vi "7. Producer Consumer Based Traffic Light Simulator.vi"() -> ()   [LabVIEW 2018]
uses:
  Typedefs/States for Producer Consumer Traffic Light.ctl
panel:
  in  "stop":bool
  out "Yellow":bool
  out "Green":bool
  out "Red":bool
  out "Traffic Lights Picture":picture
  # "Traffic Light Graphic Vector by Vecteezy\n(https://www.vecteezy.com/free-vector/graphic)"
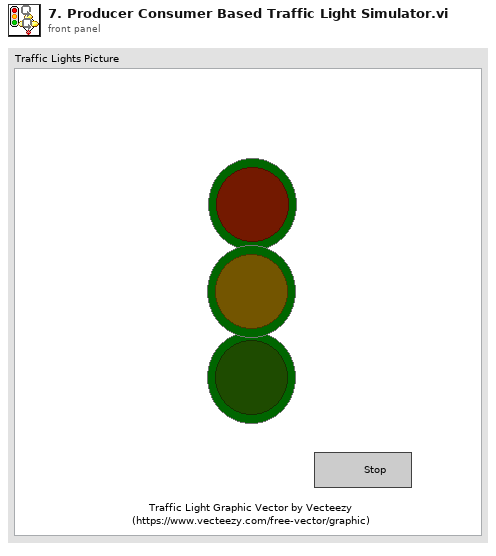
[diagram p1: front panel]
types:
  T1 = typedef "States for Producer Consumer Traffic Light.ctl" = enum16{"Red", "Yellow", "Green", "Stop"}
  T2 = cluster{"Wait Before Red":u32, "Wait Before Yellow":u32, "Wait Before Green":u32}
  T3 = cluster{"Wait Before Red":i32, "Wait Before Yellow":i32, "Wait Before Green":i32}
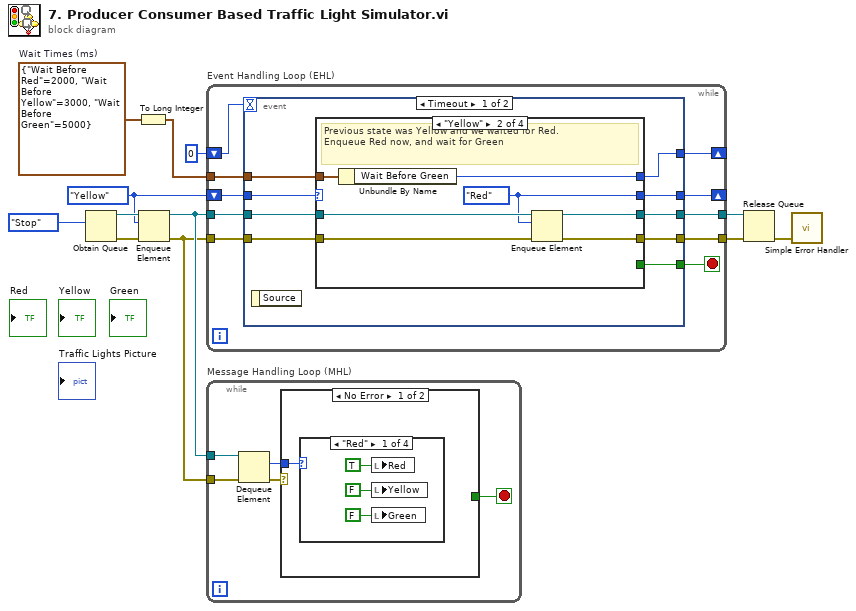
[diagram p0: block diagram]
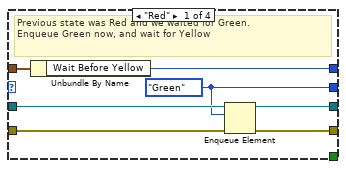
[diagram p2: hidden frame]
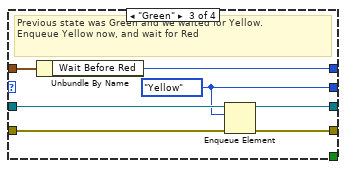
[diagram p3: hidden frame]
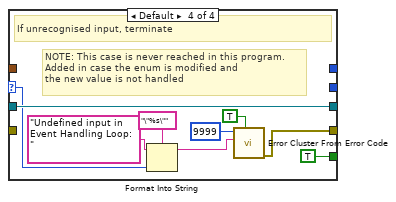
[diagram p4: hidden frame]
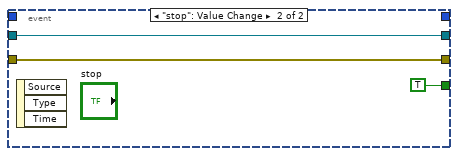
[diagram p5: hidden frame]
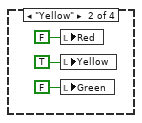
[diagram p6: hidden frame]
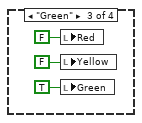
[diagram p7: hidden frame]
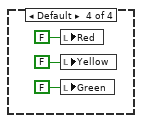
[diagram p8: hidden frame]
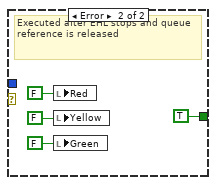
[diagram p9: hidden frame]
diagram:
  w2 = States_for_Producer_Consumer_Traffic_Light."Yellow" ("element")
  w11 = T2 {"Wait Before Red"=2000, "Wait Before Yellow"=3000, "Wait Before Green"=5000}  # Wait Times (ms)
  n1 = Obtain Queue(element data type=States_for_Producer_Consumer_Traffic_Light."Stop") -> (queue out=w12:refnum<queue>, error out=w7:errorcluster)  [unwired: 4 in, 1 out]
  n2 = To Long Integer(number=w11) -> (32bit integer=w9:T3)
  n3 = Enqueue Element(queue=w12, element=w2, error in (no error)=w7) -> (queue out=w8:refnum<queue>, error out=w6:errorcluster)  [unwired: 1 in, 1 out]
  n4 = while "Event Handling Loop (EHL)" {
    tunnel: w8 -> [w21]
    shift-right: [w16] -> _
    shift-left: w2 -> [w20]
    tunnel: w9 -> [w19]
    shift-right: [w15] -> _
    shift-left: 0 ("Wait Before Green") -> [w18]
    tunnel: [w17] -> w4
    tunnel: w6 -> [w14]
    tunnel: [w13] -> w5
    stop <- w22 stop-if-true
    n5 = event shown="[0] Timeout" {
      selector: _ -> [_ _]
      dyn-events: _ -> [_ _]
      timeout: w18 -> [_ _]
      tunnel: [w23 TRUE] -> w22
      tunnel: w21 -> [w31 w63]
      tunnel: w20 -> [w30 _]
      tunnel: w19 -> [w29 _]
      tunnel: [w28 _] -> w15
      tunnel: [w27 w63] -> w17
      tunnel: [w26 _] -> w16
      tunnel: w14 -> [w25 w62]
      tunnel: [w24 w62] -> w13
      event Timeout {
        n6 = event-data() -> ()  [unwired: 1 in, 1 out]
        n7 = case shown="\"Yellow\"" w30 {
          selector: w30 -> [_ _ _ w55]
          tunnel: w31 -> [w38 w45 w52 w61]
          tunnel: w29 -> [w37 w44 w51 _]
          tunnel: [w36 w43 w50 _] -> w28
          tunnel: [w35 w42 w49 w61] -> w27
          tunnel: [w34 w41 w48 _] -> w26
          tunnel: w25 -> [w33 w40 w47 _]
          tunnel: [w32 w39 w46 w59] -> w24
          tunnel: [_ _ _ TRUE] -> w23
          frame "Red" {
            w34 = States_for_Producer_Consumer_Traffic_Light."Green" ("element")
            # "Previous state was Red and we waited for Green.\nEnqueue Green now, and wait for Yellow"
            n8 = Unbundle By Name(w37) -> ("Wait Before Yellow"=w36:i32)
            n9 = Enqueue Element(queue=w38, element=w34, error in (no error)=w33) -> (queue out=w35:refnum<queue>, error out=w32:errorcluster)  [unwired: 1 in, 1 out]
          }
          frame "Yellow" {
            w41 = States_for_Producer_Consumer_Traffic_Light."Red" ("element")
            # "Previous state was Yellow and we waited for Red.\nEnqueue Red now, and wait for Green"
            n10 = Unbundle By Name(w44) -> ("Wait Before Green"=w43:i32)
            n11 = Enqueue Element(queue=w45, element=w41, error in (no error)=w40) -> (queue out=w42:refnum<queue>, error out=w39:errorcluster)  [unwired: 1 in, 1 out]
          }
          frame "Green" {
            w48 = States_for_Producer_Consumer_Traffic_Light."Yellow" ("element")
            # "Previous state was Green and we waited for Yellow.\nEnqueue Yellow now, and wait for Red"
            n12 = Unbundle By Name(w51) -> ("Wait Before Red"=w50:i32)
            n13 = Enqueue Element(queue=w52, element=w48, error in (no error)=w47) -> (queue out=w49:refnum<queue>, error out=w46:errorcluster)  [unwired: 1 in, 1 out]
          }
          frame Default {
            # "NOTE: This case is never reached in this program.\nAdded in case the enum is modified and\nthe new value is not handled"
            # "If unrecognised input, terminate"
            n14 = Format Into String(format string="\"%s\"", initial string="Undefined input in Event Handling Loop: " ("error message (\"\")"), w55) -> (resulting string=w54:string)  [unwired: 1 in, 1 out]
            n15 = call <vilib>:"Error Cluster From Error Code.vi"("show call chain? (False)"=TRUE, "error message (\"\")"=w54, "error code (0)"=9999) -> ("error out"=w59:errorcluster)  [unwired: 6 in]
          }
        }
      }
      event "stop": Value Change {
        n16 = event-data() -> ()  [unwired: 1 in, 3 out]
      }
    }
  }
  n17 = while "Message Handling Loop (MHL)" {
    tunnel: w8 -> [w68]
    tunnel: w6 -> [w66]
    stop <- w69 stop-if-true
    n18 = Dequeue Element(queue=w68, error in (no error)=w66) -> (element=w67:T1, error out=w65:errorcluster)  [unwired: 1 in, 2 out]
    n19 = case shown="No Error" w65 {
      tunnel: [_ TRUE] -> w69
      tunnel: w67 -> [w70 _]
      frame No Error {
        n20 = case shown="\"Red\"" w70 {
          frame "Red" {
            n21 = local write "Red"(TRUE ("Red")) -> ()
            n22 = local write "Yellow"(FALSE ("Red")) -> ()
            n23 = local write "Green"(FALSE ("Red")) -> ()
          }
          frame "Yellow" {
            n24 = local write "Red"(FALSE ("Red")) -> ()
            n25 = local write "Yellow"(TRUE ("Red")) -> ()
            n26 = local write "Green"(FALSE ("Red")) -> ()
          }
          frame "Green" {
            n27 = local write "Red"(FALSE ("Red")) -> ()
            n28 = local write "Yellow"(FALSE ("Red")) -> ()
            n29 = local write "Green"(TRUE ("Red")) -> ()
          }
          frame Default {
            n30 = local write "Red"(FALSE ("Red")) -> ()
            n31 = local write "Yellow"(FALSE ("Red")) -> ()
            n32 = local write "Green"(FALSE ("Red")) -> ()
          }
        }
      }
      frame Error {
        # "Executed after EHL stops and queue reference is released"
        n33 = local write "Red"(FALSE ("Red")) -> ()
        n34 = local write "Yellow"(FALSE ("Red")) -> ()
        n35 = local write "Green"(FALSE ("Red")) -> ()
      }
    }
  }
  n36 = Release Queue(queue=w4, error in (no error)=w5) -> (error out=w1:errorcluster)  [unwired: 1 in, 2 out]
  n37 = call <vilib>:"Simple Error Handler.vi"("error in (no error)"=w1) -> ()  [unwired: 4 in, 5 out]
